vi "FeedbackDecode_PtPtCorr.vi"(0 "Rates":sgl[](array[numeric]), 1 "Initialize":bool, 2 "Training":sgl[](array[numeric]), 3 "Lag":dbl) -> (5 "RatesLagged":dbl[](array[numeric]), 6 "TrainingLagged":dbl[](array[numeric]), 7 "Corr":dbl[](array[numeric]))   [LabVIEW 2020]
uses:
  <vilib>/Analysis/baseanly.llb/Real Outer Product.vi
  <vilib>/Analysis/NI_AALBase.lvlib
panel:
  in  "TrainBuff":dbl[][](array[numeric])
  in  "RatesBuff":dbl[][](array[numeric])
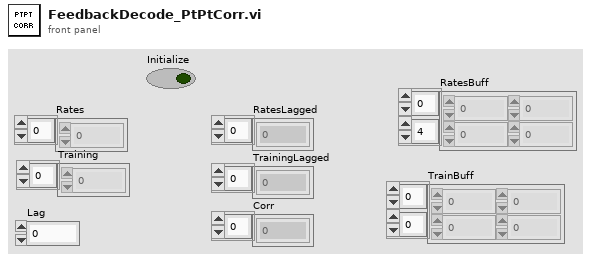
[diagram p1: front panel]
types:
  T1 = typedef "NI_Matrix.lvlib/RealMatrix.ctl" = dbl[][]
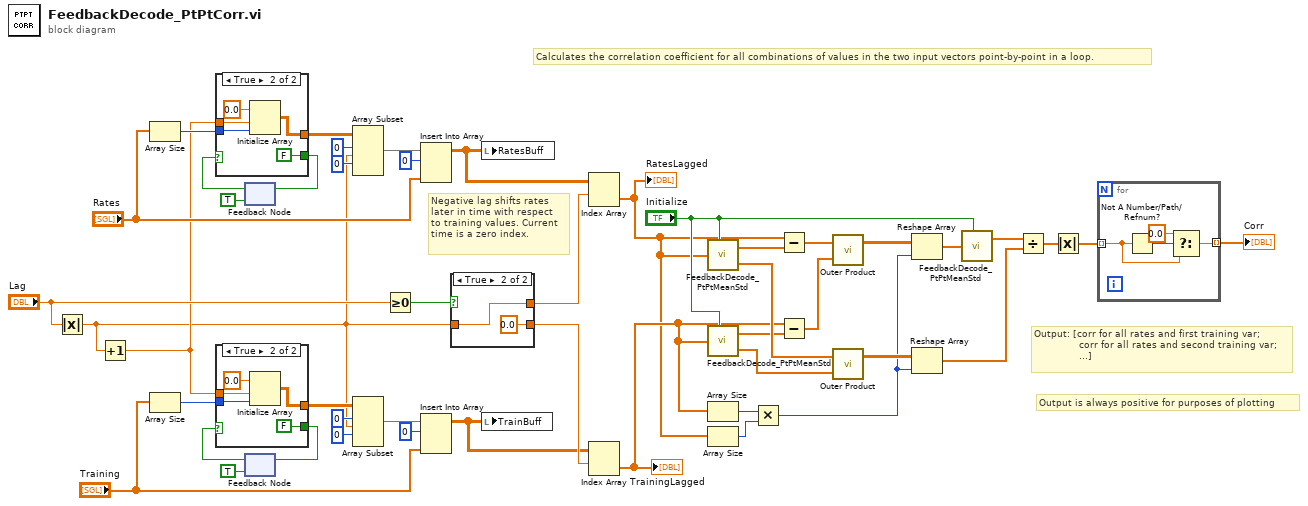
[diagram p0: block diagram]
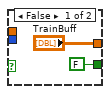
[diagram p2: hidden frame]
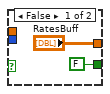
[diagram p3: hidden frame]
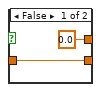
[diagram p4: hidden frame]
diagram:
  # "Output is always positive for purposes of plotting"
  # "Output: [corr for all rates and first training var;\n               corr for all rates and second training var;\n               ...]"
  # "Calculates the correlation coefficient for all combinations of values in the two input vectors point-by-point in a loop."
  # "Negative lag shifts rates\nlater in time with respect\nto training values. Current\ntime is a zero index."
  n1 = Absolute Value(x="Lag") -> (abs(x)=w1:dbl)
  n2 = Increment(x=w1) -> (x+1=w3:dbl)
  n3 = Array Size(array="Rates") -> (size(s)=w14:i32)
  n4 = Array Size(array="Training") -> (size(s)=w13:i32)
  n5 = feedback #1(TRUE) -> (w22:bool)
  n6 = case shown="True" w22 {
    tunnel: ["RatesBuff" w53] -> w20
    tunnel: [FALSE FALSE] -> w23
    tunnel: w14 -> [_ w52]
    tunnel: w3 -> [_ w51]
    frame False {
    }
    frame True {
      n7 = Initialize Array(0.0 ("element"), w51, w52) -> (w53:dbl[][])
    }
  }
  n8 = feedback-in #1(w23) -> ()
  n9 = feedback #2(TRUE) -> (w7:bool)
  n10 = case shown="True" w7 {
    tunnel: ["TrainBuff" w60] -> w9
    tunnel: [FALSE FALSE] -> w6
    tunnel: w13 -> [_ w59]
    tunnel: w3 -> [_ w58]
    frame False {
    }
    frame True {
      n11 = Initialize Array(0.0 ("element"), w58, w59) -> (w60:dbl[][])
    }
  }
  n12 = feedback-in #2(w6) -> ()
  n13 = Array Subset(array=w20, index (row)=0 ("index"), length (row)=w1, index (col)=0 ("index")) -> (w17:dbl[][])  [unwired: 1 in]
  n14 = Array Subset(array=w9, index (row)=0 ("index"), length (row)=w1, index (col)=0 ("index")) -> (w12:dbl[][])  [unwired: 1 in]
  n15 = Greater Or Equal To 0?(x="Lag") -> (x >= 0?=w35:bool)
  n16 = Insert Into Array(array=w17, index (row)=0, new element="Rates") -> (w16:dbl[][])  [unwired: 1 in]
  n17 = Insert Into Array(array=w12, index (row)=0, new element="Training") -> (w2:dbl[][])  [unwired: 1 in]
  n18 = case shown="True" w35 {
    tunnel: w1 -> [w63 w65]
    tunnel: [w63 0.0 ("Lag")] -> w33
    tunnel: [0.0 ("Lag") w65] -> w34
    frame False {
    }
    frame True {
    }
  }
  n19 = local write "RatesBuff"(w16) -> ()
  n20 = local write "TrainBuff"(w2) -> ()
  n21 = Index Array(array=w16, index (row)=w34) -> (element=w30:dbl[])  [unwired: 1 in]
  "RatesLagged" <- w30
  n22 = Index Array(array=w2, index (row)=w33) -> (element=w31:dbl[])  [unwired: 1 in]
  "TrainingLagged" <- w31
  n23 = call "FeedbackDecode_PtPtMeanStd.vi"("Initialize"="Initialize", "Array"=w30) -> ("Mean"=w45:dbl[], "Std"=w44:dbl[])  [unwired: 3 in]
  n24 = call "FeedbackDecode_PtPtMeanStd.vi"("Initialize"="Initialize", "Array"=w31) -> ("Mean"=w43:dbl[], "Std"=w42:dbl[])  [unwired: 3 in]
  n25 = Array Size(array=w31) -> (size(s)=w29:i32)
  n26 = Array Size(array=w30) -> (size(s)=w28:i32)
  n27 = Multiply(x=w29, y=w28) -> (x*y=w27:i32)
  n28 = Subtract(x=w30, y=w45) -> (x-y=w48:dbl[])
  n29 = Subtract(x=w31, y=w43) -> (x-y=w47:dbl[])
  n30 = call-poly <vilib>:"Outer Product.vi"("Y Vector"=w47, "X Vector"=w48) -> ("Outer Product"=w46:T1)  [unwired: 1 out]
  n31 = call-poly <vilib>:"Outer Product.vi"("Y Vector"=w42, "X Vector"=w44) -> ("Outer Product"=w40:T1)  [unwired: 1 out]
  n32 = Reshape Array(w46, w27) -> (w41:dbl[])
  n33 = Reshape Array(w40, w27) -> (w38:dbl[])
  n34 = call "FeedbackDecode_PtPtMeanStd.vi"("Initialize"="Initialize", "Array"=w41) -> ("Mean"=w39:dbl[])  [unwired: 3 in, 1 out]
  n35 = Divide(x=w39, y=w38) -> (x/y=w25:dbl[])
  n36 = Absolute Value(x=w25) -> (abs(x)=w26:dbl[])
  n37 = for {
    tunnel: w26 -> [w68] mode=indexing
    tunnel: [w67] -> w24 mode=indexing
    n38 = Not A Number/Path/Refnum?(number/path/refnum=w68) -> (NaN/Path/Refnum?=w70:bool)
    n39 = Select(t=0.0, s=w70, f=w68) -> (s? t:f=w67:dbl)
  }
  "Corr" <- w24
